vi "createDocument.vi"(8 "error in (no error)":errorcluster, 11 "workbook in":refnum<class "workbook.lvclass">) -> (0 "error out":errorcluster, 3 "workbook out":refnum<class "workbook.lvclass">)   [LabVIEW 2017, in "Excel_Specific.lvlib" / "workbook.lvclass"]
uses:
  workbook.lvclass
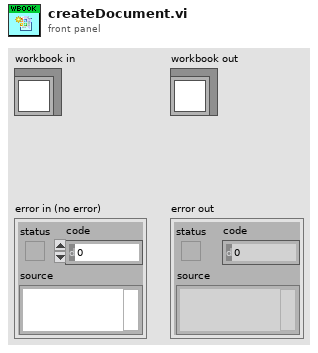
[diagram p1: front panel]
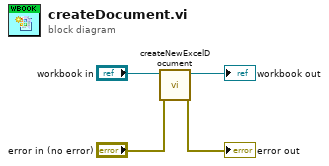
[diagram p0: block diagram]
diagram:
  n1 = call-dynamic "createNewExcelDocument.vi"("error in (no error)"="error in (no error)", "workbook in"="workbook in") -> ("error out"=→"error out":errorcluster, "workbook out"=→"workbook out":refnum<class "workbook.lvclass">)  [unwired: 8 in]
